vi "Etalon mérés dialog.vi"(8 "error in":errorcluster, 11 "Etalon név":string) -> (0 "error out":errorcluster)   [LabVIEW 2014]
panel:
  out "MainStStr":string
  in  "OK Button":bool
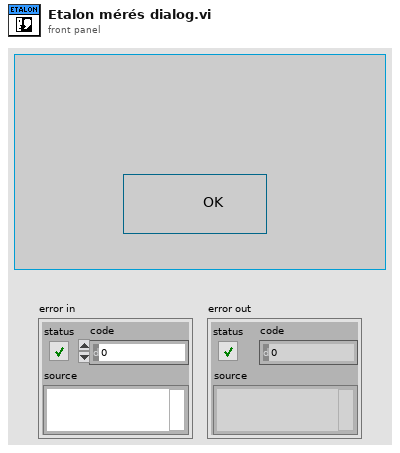
[diagram p1: front panel]
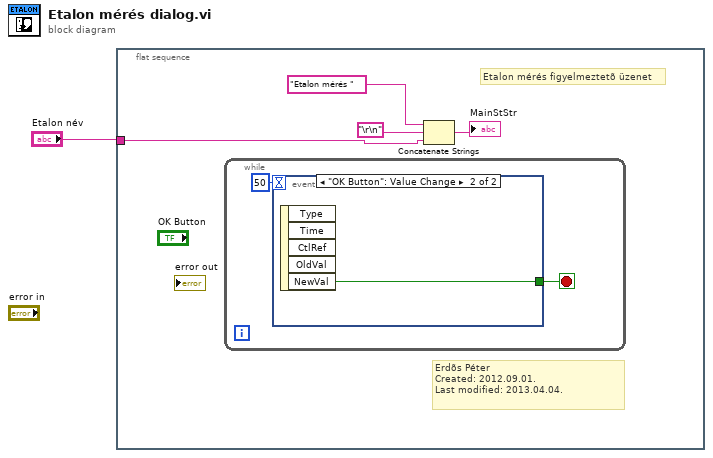
[diagram p0: block diagram]
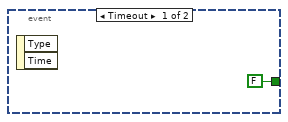
[diagram p2: hidden frame]
diagram:
  n1 = flat-sequence {
    tunnel: "Etalon név" -> [w2]
    frame #0 {
      # "Etalon mérés figyelmeztetõ üzenet"
      # "Erdõs Péter\nCreated: 2012.09.01.\nLast modified: 2013.04.04."
      n2 = while {
        stop <- w7 stop-if-true
        n3 = event shown="[1] \"OK Button\": Value Change" {
          selector: _ -> [_ _]
          dyn-events: _ -> [_ _]
          timeout: 50 -> [_ _]
          tunnel: [FALSE ("NewVal") w9] -> w7
          event Timeout {
            n4 = event-data() -> ()  [unwired: 1 in, 2 out]
          }
          event "OK Button": Value Change {
            n5 = event-data() -> ("NewVal"=w9:bool)  [unwired: 1 in, 4 out]
          }
        }
      }
      n6 = Concatenate Strings("Etalon mérés " ("MainStStr"), "\r\n", w2) -> (→"MainStStr":string)
    }
  }
